vi "Drive Direction.vi"(6 "Drive DevRef":T1={"DeviceStatus"={"status"=FALSE, "code"=0, "source"=""}, "Type"=enum."PWM", "PWM"={"PWM Channel"=enum."PWM 1", "DeadBand"={"Name"="", "maxPositivePwm"=0, "minPositivePwm"=0, "centerPwm"=0, "maxNegativePwm"=0, "minNegativePwm"=0, "angularRange"=0}}, "CAN"={"Device Number"=0, "SetOutput VI Ref"=variant(enum8{"Percent VBus", "Current", "Speed", "Position", "Voltage"} enum."Percent VBus"), "GetOutput VI Ref"=variant(refnum<k1> refnum), "Enable VI Ref"=variant(dbl 12.0), "Disable VI Ref"=variant(enum8{"Percent VBus", "Speed", "Position", "Slave", "Unchanged / Invalid", "Voltage Compensation", "Current", "Motion Profile"} enum."Percent VBus"), "Data"=variant}, "Invert"=FALSE, "DIO PWM"={"PWM \"Enable\" Channel"=enum."Invalid", "DIOChannel"=enum."Invalid", "PWM Rate"=0.0}}, 7 "Swerve DevRef":T1={"DeviceStatus"={"status"=FALSE, "code"=0, "source"=""}, "Type"=enum."PWM", "PWM"={"PWM Channel"=enum."PWM 1", "DeadBand"={"Name"="", "maxPositivePwm"=0, "minPositivePwm"=0, "centerPwm"=0, "maxNegativePwm"=0, "minNegativePwm"=0, "angularRange"=0}}, "CAN"={"Device Number"=0, "SetOutput VI Ref"=variant(enum8{"Percent VBus", "Current", "Speed", "Position", "Voltage"} enum."Percent VBus"), "GetOutput VI Ref"=variant(refnum<k1> refnum), "Enable VI Ref"=variant(dbl 12.0), "Disable VI Ref"=variant(enum8{"Percent VBus", "Speed", "Position", "Slave", "Unchanged / Invalid", "Voltage Compensation", "Current", "Motion Profile"} enum."Percent VBus"), "Data"=variant}, "Invert"=FALSE, "DIO PWM"={"PWM \"Enable\" Channel"=enum."Invalid", "DIOChannel"=enum."Invalid", "PWM Rate"=0.0}}, 9 "Module Number":enum16{"1", "2", "3", "4"}(ring), 10 "Wheel Power":dbl format="%#_13g", 11 "Desired direction (radians)":dbl=6.283185307179586 format="%#_13g") -> (2 "Sensor Position":dbl, 3 "setpoint":dbl format="%#_13g")   [LabVIEW 2017, in "Huskie Swerve.lvlib"]
uses:
  Huskie Swerve.lvlib
  <vilib>/Rock Robotics/WPI/MotorControl/WPI_MotorControlDeviceRef.ctl
  <vilib>/Rock Robotics/WPI/MotorControl/WPI_MotorControlType.ctl
  <vilib>/Rock Robotics/SystemInterfaces/DIO/FPGA_DIOPWMChannel.ctl
  <vilib>/Rock Robotics/WPI/PWM/WPI_PWMDeadband.ctl
  <vilib>/Rock Robotics/SystemInterfaces/DIO/FPGA_DIOChannel.ctl
  Public/Documents/Cross The Road Electronics/Phoenix-LabVIEW/Motor Controller/Controls/CTRE_Phoenix_MotorControl_ControlMode.ctl
  Public/Documents/Cross The Road Electronics/Phoenix-LabVIEW/Motor Controller/Get/CTRE_Phoenix_MotorController_GetSelectedSensorData.vi
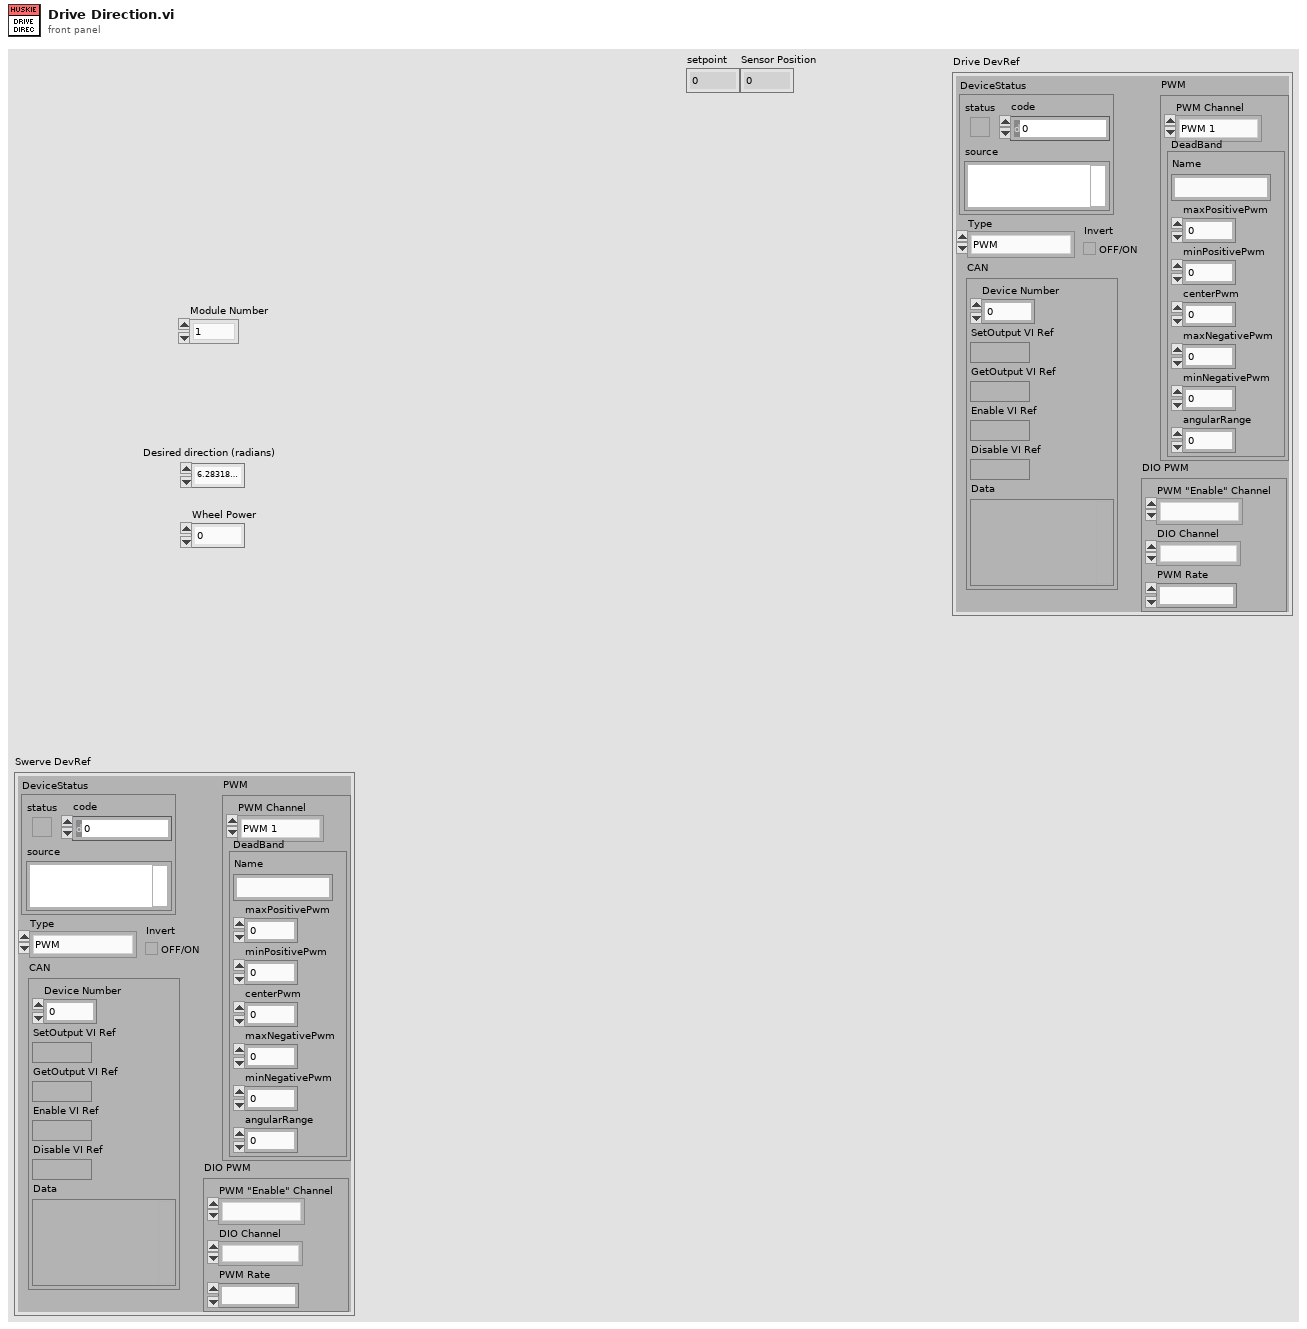
[diagram p1: front panel]
types:
  T1 = typedef "WPI_MotorControlDeviceRef.ctl" = cluster{"DeviceStatus":errorcluster, "Type":T2, "PWM":cluster{"PWM Channel":T3, "DeadBand":T4}, "CAN":cluster{"Device Number":u8, "SetOutput VI Ref":variant, "GetOutput VI Ref":variant, "Enable VI Ref":variant, "Disable VI Ref":variant, "Data":variant}, "Invert":bool, "DIO PWM":cluster{"PWM \"Enable\" Channel":T3, "DIOChannel":T5, "PWM Rate":dbl}}
  T2 = typedef "WPI_MotorControlType.ctl" = enum16{"PWM", "CAN", "DIO PWM"}
  T3 = typedef "FPGA_DIOPWMChannel.ctl" = enum8{"PWM 0", "PWM 1", "PWM 2", "PWM 3", "PWM 4", "PWM 5", "PWM 6", "PWM 7", "PWM 8", "PWM 9", "PWM MXP 0", "PWM MXP 1", "PWM MXP 2", "PWM MXP 3", "PWM MXP 4", "PWM MXP 5", "PWM MXP 6", "PWM MXP 7", "PWM MXP 8", "PWM MXP 9", "Invalid"}
  T4 = typedef "WPI_PWMDeadband.ctl" = cluster{"Name":string, "maxPositivePwm":i32, "minPositivePwm":i32, "centerPwm":i32, "maxNegativePwm":i32, "minNegativePwm":i32, "angularRange":u16}
  T5 = typedef "FPGA_DIOChannel.ctl" = enum8{"DIO 0", "DIO 1", "DIO 2", "DIO 3", "DIO 4", "DIO 5", "DIO 6", "DIO 7", "DIO 8", "DIO 9", "DIO MXP 0", "DIO MXP 1", "DIO MXP 2", "DIO MXP 3", "DIO MXP 4", "DIO MXP 5", "DIO MXP 6", "DIO MXP 7", "DIO MXP 8", "DIO MXP 9", "DIO MXP 10", "DIO MXP 11", "DIO MXP 12", "DIO MXP 13", "DIO MXP 14", "DIO MXP 15", "SPI Port CS1", "SPI Port CS2", "SPI Port CS3", "SPI Port MISO", "SPI Port MOSI", "Invalid"}
  T6 = typedef "CTRE_Phoenix_MotorControl_ControlMode.ctl" = u16
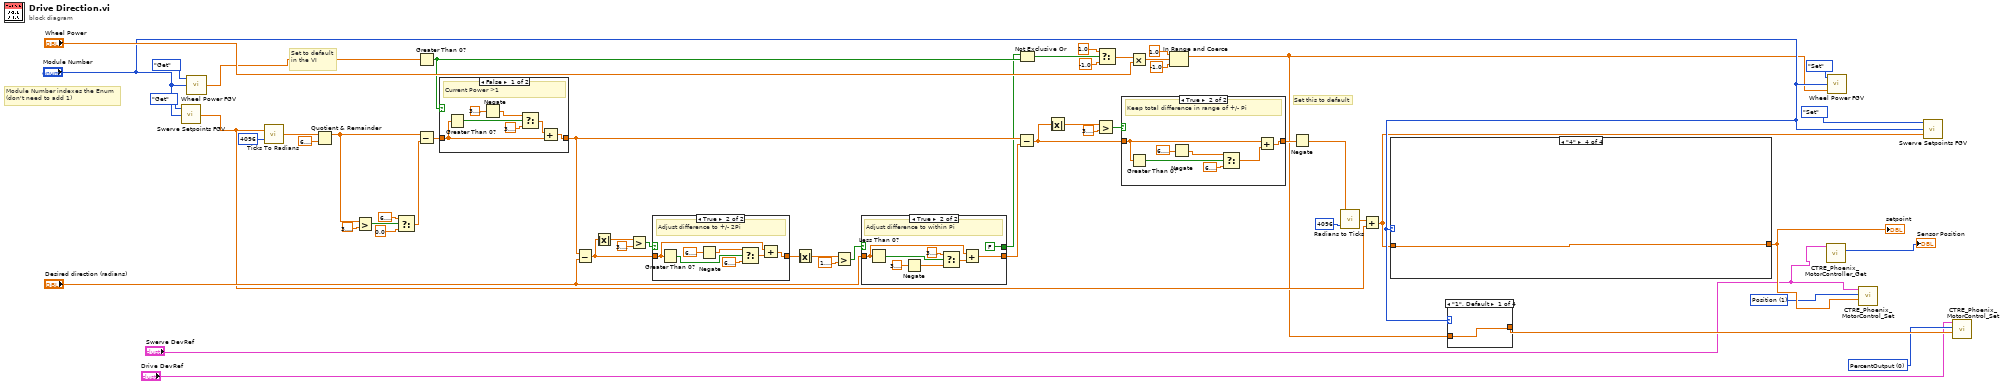
[diagram p0: block diagram]
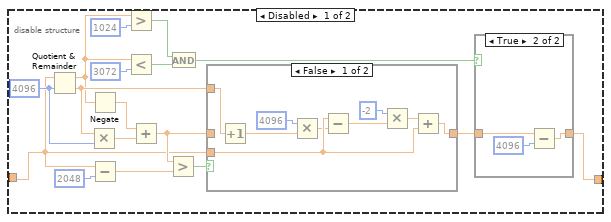
[diagram p7: hidden frame]
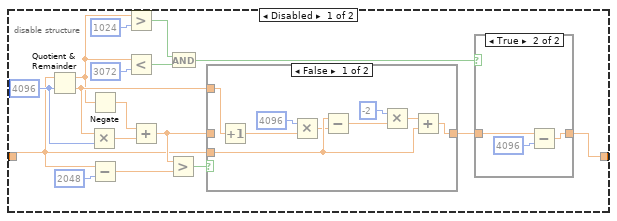
[diagram p11: hidden frame]
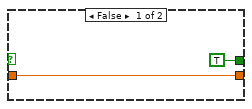
[diagram p15: hidden frame]
diagram:
  w3 = T6 0 items=["PercentOutput"=0, "Position"=1, "Velocity"=2, "Current"=3, "Follower"=5, "MotionProfile"=6, "MotionMagic"=7, "MotionMagicArc"=8, "MotionProfileArc"=10, "Disabled"=15] ("Control Mode")
  w6 = T6 1 items=["PercentOutput"=0, "Position"=1, "Velocity"=2, "Current"=3, "Follower"=5, "MotionProfile"=6, "MotionMagic"=7, "MotionMagicArc"=8, "MotionProfileArc"=10, "Disabled"=15] ("Control Mode")
  # "Module Number indexes the Enum\n(don't need to add 1)"
  # "Set this to default"
  # "Set to default\nin the VI"
  n1 = call "Swerve Setpoints FGV.vi"("Swerve Number"="Module Number", "Action"=enum16{"Set", "Get"}."Get") -> ("Setpoint"=w15:dbl)  [unwired: 1 in]
  n2 = call "Wheel Power FGV.vi"("Swerve Number"="Module Number", "Action"=enum16{"Set", "Get"}."Get") -> ("Power"=w16:dbl)  [unwired: 1 in]
  n3 = call "Ticks To Radians.vi"("Ticks/Rev"=4096, "Ticks"=w15) -> ("Radians"=w48:dbl)
  n4 = Quotient & Remainder(x=w48, y=6.283185307179586) -> (x-y*floor(x/y)=w46:dbl)  [unwired: 1 out]
  n5 = Greater?(x=w46, y=3.141592653589793) -> (0:w52:bool)
  n6 = Select(t=6.283185307179586, s=w52, f=0.0) -> (s? t:f=w49:dbl)
  n7 = Greater Than 0?(x=w16) -> (x > 0?=w18:bool)
  n8 = Subtract(x=w46, y=w49) -> (x-y=w47:dbl)
  n9 = case shown="False" w18 {
    tunnel: w47 -> [w57 w63]
    tunnel: [w56 w63] -> w30
    frame False {
      # "Current Power >1"
      n10 = Greater Than 0?(x=w57) -> (x > 0?=w62:bool)
      n11 = Negate(x=3.141592653589793) -> (-x=w61:dbl)
      n12 = Select(t=w61, s=w62, f=3.141592653589793) -> (s? t:f=w58:dbl)
      n13 = Add(x=w58, y=w57) -> (x+y=w56:dbl)
    }
    frame True {
      # "Current Power >1"
    }
  }
  n14 = Subtract(x=w30, y="Desired direction (radians)") -> (x-y=w42:dbl)
  n15 = Absolute Value(x=w42) -> (abs(x)=w43:dbl)
  n16 = Greater?(x=w43, y=3.141592653589793) -> (0:w45:bool)
  n17 = case shown="True" w45 {
    tunnel: w42 -> [w64 w66]
    tunnel: [w64 w65] -> w39
    frame False {
    }
    frame True {
      # "Adjust difference to +/- 2Pi"
      n18 = Greater Than 0?(x=w66) -> (x > 0?=w71:bool)
      n19 = Negate(x=6.283185307179586) -> (-x=w68:dbl)
      n20 = Select(t=w68, s=w71, f=6.283185307179586) -> (s? t:f=w67:dbl)
      n21 = Add(x=w66, y=w67) -> (x+y=w65:dbl)
    }
  }
  n22 = Absolute Value(x=w39) -> (abs(x)=w40:dbl)
  n23 = Greater?(x=w40, y=1.5707963267948966) -> (0:w38:bool)
  n24 = case shown="True" w38 {
    tunnel: "Desired direction (radians)" -> [w73 w76]
    tunnel: [w73 w75] -> w31
    tunnel: [TRUE FALSE] -> w17
    frame False {
    }
    frame True {
      # "Adjust difference to within Pi"
      n25 = Less Than 0?(x=w76) -> (x < 0?=w81:bool)
      n26 = Negate(x=3.141592653589793) -> (-x=w78:dbl)
      n27 = Select(t=3.141592653589793, s=w81, f=w78) -> (s? t:f=w77:dbl)
      n28 = Add(x=w76, y=w77) -> (x+y=w75:dbl)
    }
  }
  n29 = Subtract(x=w30, y=w31) -> (x-y=w33:dbl)
  n30 = Not Exclusive Or(1:w18, 2:w17) -> (0:w26:bool)
  n31 = Absolute Value(x=w33) -> (abs(x)=w36:dbl)
  n32 = Greater?(x=w36, y=3.141592653589793) -> (0:w35:bool)
  n33 = Select(t=1.0, s=w26, f=-1.0 ("t")) -> (s? t:f=w23:dbl)
  n34 = case shown="True" w35 {
    tunnel: w33 -> [w82 w84]
    tunnel: [w82 w83] -> w32
    frame False {
    }
    frame True {
      # "Keep total difference in range of +/- Pi"
      n35 = Greater Than 0?(x=w84) -> (x > 0?=w89:bool)
      n36 = Negate(x=6.283185307179586) -> (-x=w87:dbl)
      n37 = Select(t=w87, s=w89, f=6.283185307179586) -> (s? t:f=w86:dbl)
      n38 = Add(x=w84, y=w86) -> (x+y=w83:dbl)
    }
  }
  n39 = Multiply(x=w23, y="Wheel Power") -> (x*y=w19:dbl)
  n40 = In Range and Coerce(upper limit=1.0, x=w19, lower limit=-1.0) -> (coerced(x)=w9:dbl)  [unwired: 1 out]
  n41 = Negate(x=w32) -> (-x=w29:dbl)
  n42 = call "Radians to Ticks.vi"("Ticks/rev"=4096, "Radians"=w29) -> ("Ticks"=w27:dbl)
  n43 = Add(x=w27, y=w15) -> (x+y=w8:dbl)
  n44 = case shown="\"4\"" "Module Number" {
    tunnel: w8 -> [w90 w92 w126 w159]
    tunnel: [w90 w91 w125 w159] -> w7
    frame "1", Default {
    }
    frame "2" {
      n45 = disable-structure shown="Enabled" {
        disable-tunnel: w92 -> [w93 w124]
        disable-tunnel: [w94 w124] -> w91
        frame Disabled {
          w109 = 4096
          n46 = Quotient & Remainder(x=w93, y=w109) -> (x-y*floor(x/y)=w99:dbl, floor(x/y)=w102:dbl)
          n47 = Multiply(x=w102, y=w109) -> (x*y=w103:dbl)
          n48 = Negate(x=w99) -> (-x=w108:dbl)
          n49 = Subtract(x=w93, y=2048) -> (x-y=w106:dbl)
          n50 = Greater?(x=w99, y=1024) -> (0:w96:bool)
          n51 = Less?(x=w99, y=3072) -> (x < y?=w97:bool)
          n52 = Add(x=w108, y=w103) -> (x+y=w104:dbl)
          n53 = Greater?(x=w104, y=w106) -> (0:w105:bool)
          n54 = And(x=w96, y=w97) -> (x .and. y?=w95:bool)
          n55 = case shown="False" w105 {
            tunnel: w104 -> [_ w123]
            tunnel: [w119 w123] -> w101
            tunnel: w93 -> [w118 _]
            tunnel: w102 -> [w117 _]
            frame False {
              n56 = Increment(x=w117) -> (x+1=w115:dbl)
              n57 = Multiply(x=4096, y=w115) -> (x*y=w114:dbl)
              n58 = Subtract(x=w118, y=w114) -> (x-y=w122:dbl)
              n59 = Multiply(x=-2, y=w122) -> (x*y=w120:dbl)
              n60 = Add(x=w120, y=w118) -> (x+y=w119:dbl)
            }
            frame True {
            }
          }
          n61 = case shown="True" w95 {
            tunnel: w101 -> [w110 w112]
            tunnel: [w110 w111] -> w94
            frame False {
            }
            frame True {
              n62 = Subtract(x=w112, y=4096) -> (x-y=w111:dbl)
            }
          }
        }
        frame Enabled {
        }
      }
    }
    frame "3" {
      n63 = disable-structure shown="Enabled" {
        disable-tunnel: w126 -> [w127 w158]
        disable-tunnel: [w128 w158] -> w125
        frame Disabled {
          w143 = 4096
          n64 = Quotient & Remainder(x=w127, y=w143) -> (x-y*floor(x/y)=w133:dbl, floor(x/y)=w136:dbl)
          n65 = Multiply(x=w136, y=w143) -> (x*y=w137:dbl)
          n66 = Negate(x=w133) -> (-x=w142:dbl)
          n67 = Subtract(x=w127, y=2048) -> (x-y=w140:dbl)
          n68 = Greater?(x=w133, y=1024) -> (0:w130:bool)
          n69 = Less?(x=w133, y=3072) -> (x < y?=w131:bool)
          n70 = Add(x=w142, y=w137) -> (x+y=w138:dbl)
          n71 = Greater?(x=w138, y=w140) -> (0:w139:bool)
          n72 = And(x=w130, y=w131) -> (x .and. y?=w129:bool)
          n73 = case shown="False" w139 {
            tunnel: w138 -> [_ w157]
            tunnel: [w153 w157] -> w135
            tunnel: w127 -> [w152 _]
            tunnel: w136 -> [w151 _]
            frame False {
              n74 = Increment(x=w151) -> (x+1=w149:dbl)
              n75 = Multiply(x=4096, y=w149) -> (x*y=w148:dbl)
              n76 = Subtract(x=w152, y=w148) -> (x-y=w156:dbl)
              n77 = Multiply(x=-2, y=w156) -> (x*y=w154:dbl)
              n78 = Add(x=w154, y=w152) -> (x+y=w153:dbl)
            }
            frame True {
            }
          }
          n79 = case shown="True" w129 {
            tunnel: w135 -> [w144 w146]
            tunnel: [w144 w145] -> w128
            frame False {
            }
            frame True {
              n80 = Subtract(x=w146, y=4096) -> (x-y=w145:dbl)
            }
          }
        }
        frame Enabled {
        }
      }
    }
    frame "4" {
    }
  }
  "setpoint" <- w7
  n81 = case shown="\"1\", Default" "Module Number" {
    tunnel: w9 -> [w160 w161 w162 w163]
    tunnel: [w160 w161 w162 w163] -> w4
    frame "1", Default {
    }
    frame "2" {
    }
    frame "3" {
    }
    frame "4" {
    }
  }
  n82 = call-poly "CTRE_Phoenix_MotorController_Get.vi"("PhoenixMotorControlDevRef"="Swerve DevRef") -> ("Position (Raw Sensor Units)"=→"Sensor Position":i32)  [unwired: 11 in, 3 out]
  n83 = call "Wheel Power FGV.vi"("New Power"=w9, "Swerve Number"="Module Number", "Action"=enum16{"Set", "Get"}."Set") -> ()  [unwired: 1 out]
  n84 = call "CTRE_Phoenix_MotorControl_Set.vi"("Output"=w7, "Control Mode"=w6, "PhoenixMotorControlDevRef"="Swerve DevRef") -> ()  [unwired: 7 in, 2 out]
  n85 = call "Swerve Setpoints FGV.vi"("New Setpoint"=w8, "Swerve Number"="Module Number", "Action"=enum16{"Set", "Get"}."Set") -> ()  [unwired: 1 out]
  n86 = call "CTRE_Phoenix_MotorControl_Set.vi"("Output"=w4, "Control Mode"=w3, "PhoenixMotorControlDevRef"="Drive DevRef") -> ()  [unwired: 7 in, 2 out]
